vi "Scan Project For Item By Name.vi"(0 "ProjectItem in":refnum<vi>, 5 "Type":string, 7 "Item Name":string, 11 "error in (no error)":errorcluster) -> (4 "ProjectItem out":refnum<vi>, 6 "Found":bool, 15 "error out":errorcluster)   [LabVIEW 2020, in "MVA Message Mapper.lvlib"]
uses:
  <vilib>/gpm_packages/@cs/Bus-message-mapper/Source/MVA Message Mapper.lvlib
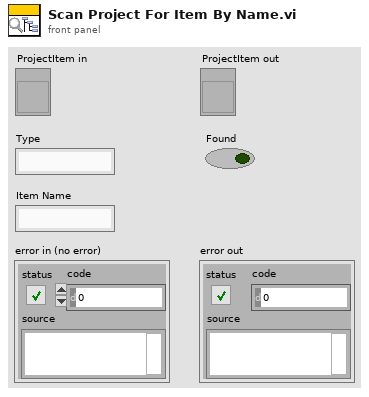
[diagram p1: front panel]
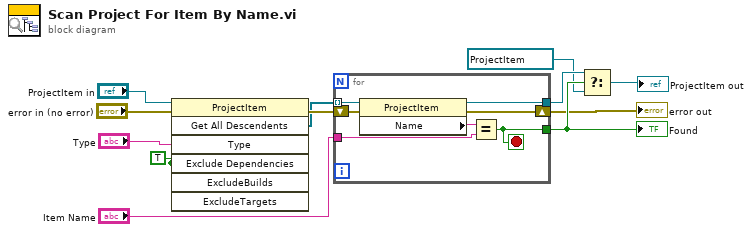
[diagram p0: block diagram]
diagram:
  w3 = TRUE ("ExcludeDependencies")
  n1 = invoke on="Invoke Node" class="ProjectItem" method="Get All Descendents"(reference="ProjectItem in", error in="error in (no error)", "Type"="Type", "Exclude Dependencies"=w3, "ExcludeBuilds"=w3) -> (error out=w8:errorcluster, "All Descendents"=w2:refnum<vi>[])  [unwired: 2 in, 5 out]
  n2 = for {
    tunnel: w2 -> [w19] mode=indexing
    tunnel: "Item Name" -> [w18]
    tunnel: [w16] -> w10
    tunnel: [w15] -> w11
    shift-right: [w14] -> w7
    shift-left: w8 -> [w13]
    stop <- w15 stop-if-true
    n3 = property class="ProjectItem"(reference=w19, error in=w13) -> (reference out=w16:refnum<vi>, error out=w14:errorcluster, "Name"=w17:string)
    n4 = Equal?(x=w17, y=w18) -> (x = y?=w15:bool)
  }
  "Found" <- w11
  "error out" <- w7
  n5 = Select(t=w10, s=w11, f=refnum<vi> refnum) -> (s? t:f=→"ProjectItem out":refnum<vi>)
